vi "Write_Buffer_To_Log.vi"(8 "error in":errorcluster) -> (0 "error out":errorcluster)   [LabVIEW 2017]
uses:
  frc-software-2018/SwerveLibrary/Huskie Board.ctl
  frc-software-2018/SwerveLibrary/Refname to String (Huskie Board).vi
  frc-software-2018/SwerveLibrary/Huskie Swerve.lvlib
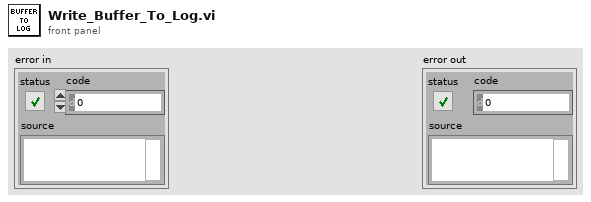
[diagram p1: front panel]
types:
  T1 = typedef "Huskie Swerve.lvlib/Huskie Board.ctl" = enum16{"Huskie Board", "Log Queue", ""}
  T2 = typedef "WPI_SerialPortRef.ctl" = cluster{"DevStatus":errorcluster, "Serial Port Name":refnum<visa-resource-name>}
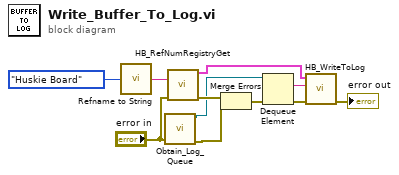
[diagram p0: block diagram]
diagram:
  n1 = call-poly "Refname to String.vi"("Enum"=Huskie_Board."Huskie Board") -> ("resulting string"=w10:string)
  n2 = call "Obtain_Log_Queue.vi"("error in"="error in") -> ("error out"=w1:errorcluster, "queue out"=w2:refnum<queue>)  [unwired: 9 in]
  n3 = call <vilib>:"HB_RefNumRegistryGet.vi"("refnum name"=w10, "error in (no error)"="error in") -> ("HBDevRef"=w9:T2, "error out"=w6:errorcluster)  [unwired: 12 in]
  n4 = Merge Errors(w6, w1) -> (w7:errorcluster)
  n5 = Dequeue Element(queue=w2, error in (no error)=w7) -> (element=w8:string, error out=w5:errorcluster)  [unwired: 1 in, 2 out]
  n6 = call <vilib>:"HB_WriteToLog.vi"("error in (no error)"=w5, "Log string"=w8, "HBDevRef"=w9) -> ("error out"=→"error out":errorcluster)  [unwired: 7 in, 1 out]
